vi "HCC Individual Cycle Conditions.vi"(8 "Error In":errorcluster, 9 "Total Cycle Count (Current)":u16, 10 "Input Cycle Count":u16, 11 "Conditions in":T1) -> (0 "Error Out":errorcluster, 1 "Reset Timer":bool, 2 "Enter Timer Loop":bool, 3 "Conditions out":T1, 4 "Timer Limit":dbl, 5 "Stop Loop":bool)   [LabVIEW 2016]
uses:
  Type Definitions/HCC Cycle Check Conditions.ctl
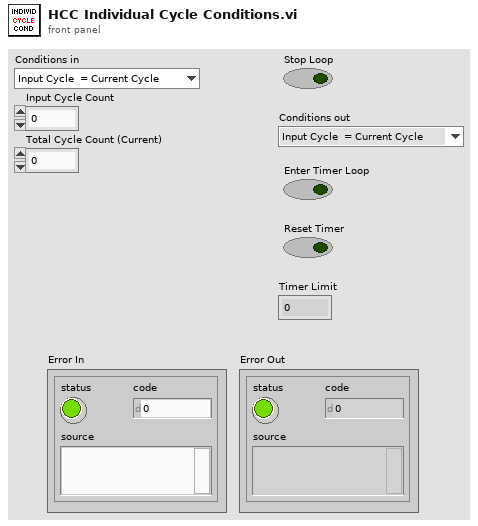
[diagram p1: front panel]
types:
  T1 = typedef "HCC Cycle Check Conditions.ctl" = enum16{"Input Cycle  = Current Cycle", "Input Cycle = 1-Current Cycle", "Input Cycle = 1+Current Cycle", "Input Cycle = <1-Current Cycle", "Input Cycle = >1+Current Cycle"}
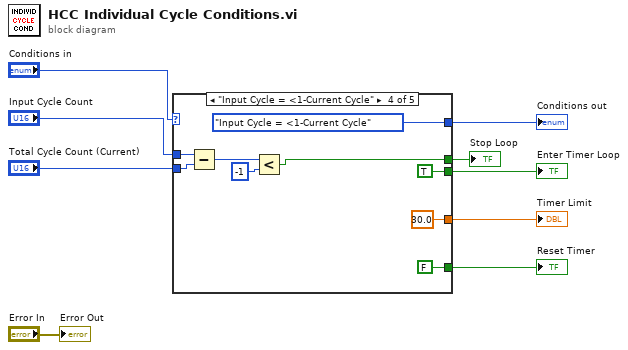
[diagram p0: block diagram]
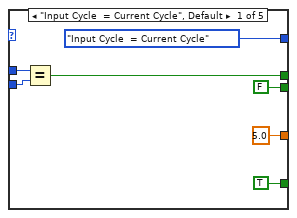
[diagram p2: hidden frame]
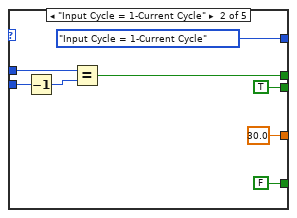
[diagram p3: hidden frame]
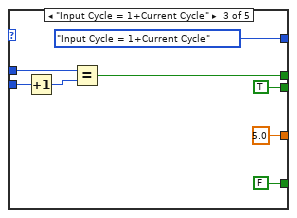
[diagram p4: hidden frame]
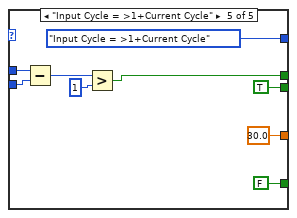
[diagram p5: hidden frame]
diagram:
  n1 = case shown="\"Input Cycle = <1-Current Cycle\"" "Conditions in" {
    tunnel: "Input Cycle Count" -> [w16 w18 w27 w37 w44]
    tunnel: "Total Cycle Count (Current)" -> [w15 w20 w28 w36 w43]
    tunnel: [w14 w17 w25 w33 w42] -> w5
    tunnel: [HCC_Cycle_Check_Conditions."Input Cycle  = Current Cycle" ("Conditions") HCC_Cycle_Check_Conditions."Input Cycle = 1-Current Cycle" ("Conditions") HCC_Cycle_Check_Conditions."Input Cycle = 1+Current Cycle" ("Conditions") HCC_Cycle_Check_Conditions."Input Cycle = <1-Current Cycle" ("Conditions") HCC_Cycle_Check_Conditions."Input Cycle = >1+Current Cycle" ("Conditions")] -> w6
    tunnel: [FALSE ("Enter Timer Loop") TRUE ("Enter Timer Loop") TRUE ("Enter Timer Loop") TRUE ("Enter Timer Loop") TRUE ("Enter Timer Loop")] -> w7
    tunnel: [TRUE ("Enter Timer Loop") FALSE ("Enter Timer Loop") FALSE ("Enter Timer Loop") FALSE ("Enter Timer Loop") FALSE ("Enter Timer Loop")] -> w8
    tunnel: [5.0 ("Timer Limit") 30.0 ("Timer Limit") 5.0 ("Timer Limit") 30.0 ("Timer Limit") 30.0 ("Timer Limit")] -> w9
    frame "Input Cycle  = Current Cycle", Default {
      n2 = Equal?(x=w16, y=w15) -> (x = y?=w14:bool)
    }
    frame "Input Cycle = 1-Current Cycle" {
      n3 = Decrement(x=w20) -> (x-1=w19:u16)
      n4 = Equal?(x=w18, y=w19) -> (x = y?=w17:bool)
    }
    frame "Input Cycle = 1+Current Cycle" {
      n5 = Increment(x=w28) -> (x+1=w26:u16)
      n6 = Equal?(x=w27, y=w26) -> (x = y?=w25:bool)
    }
    frame "Input Cycle = <1-Current Cycle" {
      n7 = Subtract(x=w37, y=w36) -> (x-y=w35:u16)
      n8 = Less?(x=w35, y=-1) -> (x < y?=w33:bool)
    }
    frame "Input Cycle = >1+Current Cycle" {
      n9 = Subtract(x=w44, y=w43) -> (x-y=w46:u16)
      n10 = Greater?(x=w46, y=u16 1) -> (0:w42:bool)
    }
  }
  "Timer Limit" <- w9
  "Reset Timer" <- w8
  "Enter Timer Loop" <- w7
  "Conditions out" <- w6
  "Stop Loop" <- w5
  "Error Out" <- "Error In"
